vi "GetCursorData.vi"(6 "Value":u16, 9 "CrsrList":T1, 10 "X軸名称[]":string[](array[string]), 11 "Y軸名称[]":string[](array[string])) -> (1 "Index":i32, 3 "カーソルデータ":T2)   [LabVIEW 2014]
uses:
  <vilib>/Utility/miscctls.llb/LVCursorListTypeDef.ctl
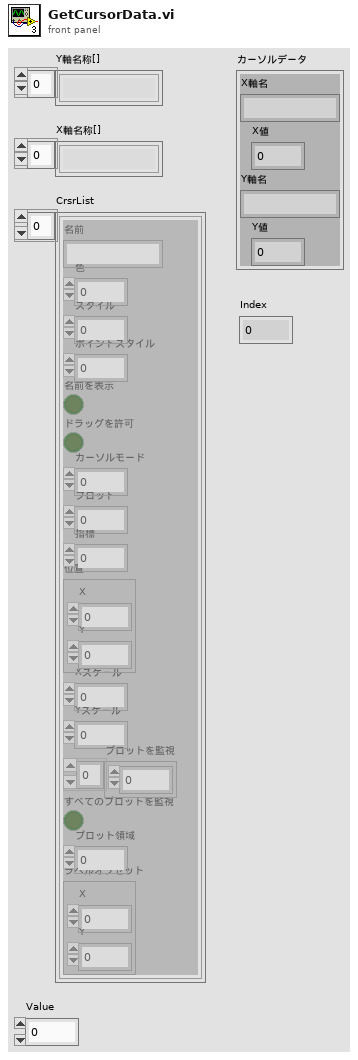
[diagram p1: front panel]
types:
  T1 = typedef "LVCursorListTypeDef.ctl" = cluster{"Name":string, "Color":u32, "Style":u8, "Point Style":u8, "Name Visible":bool, "Allow Drag":bool, "Cursor Mode":u32, "Plot":i32, "Index":i32, "Position":cluster{"X":dbl, "Y":dbl}, "X Scale":u32, "Y Scale":u32, "Watch Plots":i32[], "Watch All Plots":bool, "Plot Area":i32, "Label Offset":cluster{"X":dbl, "Y":dbl}}[]
  T2 = cluster{"X軸名":string, "X値":dbl, "Y軸名":string, "Y値":dbl}
  T3 = cluster{"Name":string, "Color":u32, "Style":u8, "Point Style":u8, "Name Visible":bool, "Allow Drag":bool, "Cursor Mode":u32, "Plot":i32, "Index":i32, "Position":cluster{"X":dbl, "Y":dbl}, "X Scale":u32, "Y Scale":u32, "Watch Plots":i32[], "Watch All Plots":bool, "Plot Area":i32, "Label Offset":cluster{"X":dbl, "Y":dbl}}
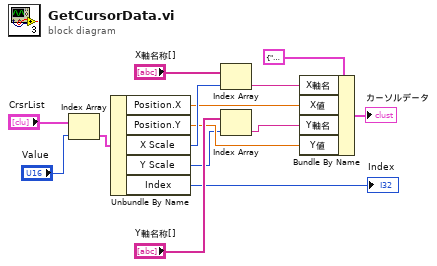
[diagram p0: block diagram]
diagram:
  n1 = Index Array(array="CrsrList", index="Value") -> (element=w3:T3)
  n2 = Unbundle By Name(w3) -> ("Position.X"=w8:dbl, "Position.Y"=w7:dbl, "X Scale"=w10:u32, "Y Scale"=w4:u32, "Index"=→"Index":i32)
  n3 = Index Array(array="X軸名称[]", index=w10) -> (element=w11:string)
  n4 = Index Array(array="Y軸名称[]", index=w4) -> (element=w6:string)
  n5 = Bundle By Name(cluster=T2 {"X軸名"="X軸名", "X値"=0.30000000000000004, "Y軸名"="Y軸名", "Y値"=3782.085818} ("クラスタ"), "X軸名"=w11, "X値"=w8, "Y軸名"=w6, "Y値"=w7) -> (→"カーソルデータ":T2)
